vi "Item Names.get.vi"(8 "error in (no error)":errorcluster, 11 "selection_dropdown in":refnum<class "selection_dropdown.lvclass">) -> (0 "error out":errorcluster, 2 "Item Names":string[](array[string]), 3 "selection_dropdown out":refnum<class "selection_dropdown.lvclass">)   [LabVIEW 2024, in "selection_dropdown.lvclass"]
uses:
  selection_dropdown.lvclass
  selection_dropdown.lvclass/selection_dropdown.ctl
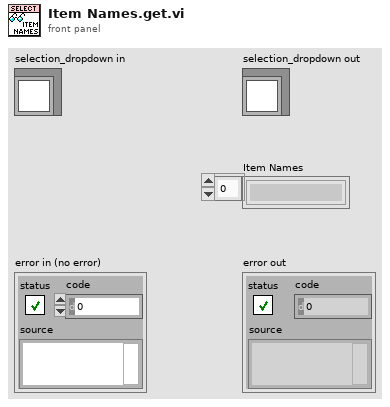
[diagram p1: front panel]
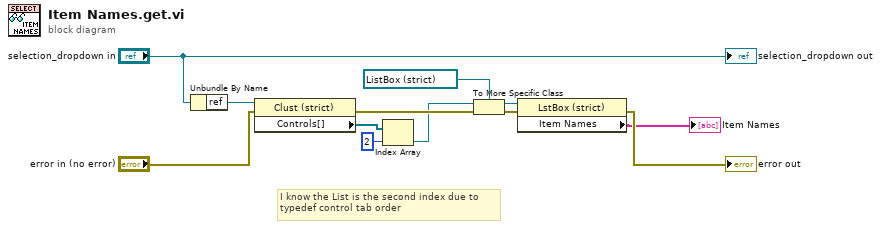
[diagram p0: block diagram]
diagram:
  # "I know the List is the second index due to \ntypedef control tab order"
  n1 = Unbundle By Name("selection_dropdown in") -> ("ref"=w11:refnum<vi>)
  n2 = property class="Clust (strict)"(reference=w11, error in="error in (no error)") -> (error out=w8:errorcluster, "Controls[]"=w10:refnum<vi>[])  [unwired: 1 out]
  n3 = Index Array(array=w10, index=2) -> (element=w6:refnum<vi>)
  n4 = To More Specific Class(target class=refnum<vi> refnum ("Listbox"), reference=w6, error in=w8) -> (specific class reference=w5:refnum<vi>, error out=w7:errorcluster)
  n5 = property class="LstBox (strict)"(reference=w5, error in=w7) -> (error out=→"error out":errorcluster, "Item Names"=→"Item Names":string[])  [unwired: 1 out]
  "selection_dropdown out" <- "selection_dropdown in"
